vi "Accel calib routine.vi"(6 "Connection Status":T1={"MAC Address"="", "cnx handle"=0, "cnx flags"=0, "Address Type"=125, "Connection Interval (ms)"=125, "Timeout(ms)"=125, "Latency"=0, "bonding handle"=0} {"Address Type" items=["Public", "Random"]}, 8 "Error In":errorcluster, 11 "VISA resource in":refnum<visa-resource-name>) -> ()   [LabVIEW 2016]
uses:
  <vilib>/BLE/type_def/connection_status_bundle.ctl
  <vilib>/BLE/type_def/address_type.ctl
  Typedef/Accel calib - States.ctl
  Typedef/BLE char handle.ctl
  Typedef/Accel FSR.ctl
  <vilib>/Analysis/baseanly.llb/Mean (DBL).vi
  <vilib>/BLE/ble_functions/ble_write_by_handle_uint8array.vi
  <vilib>/Analysis/NI_AALBase.lvlib
panel:
  in  "Set & Save":bool
  in  "Exit":bool
  in  "Next":bool
  out "Calibration results":i32(listbox)
  out "Instructions":string="Press START CALIBRATION to calibrate the accelerometer"
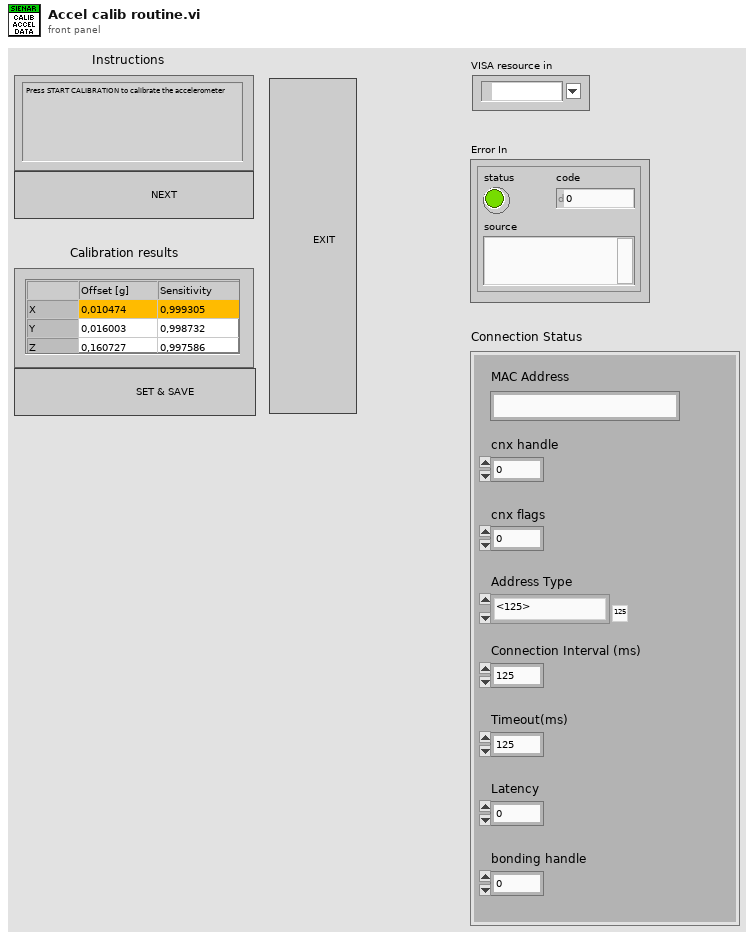
[diagram p1: front panel]
types:
  T1 = typedef "connection_status_bundle.ctl" = cluster{"MAC Address":string, "cnx handle":u8, "cnx flags":u8, "Address Type":T2, "Connection Interval (ms)":u16, "Timeout(ms)":u16, "Latency":u16, "bonding handle":u8}
  T2 = typedef "address_type.ctl" = u8
  T3 = typedef "Accel calib - States.ctl" = enum16{"Start calibration", "Acquire X+", "Acquire X-", "Acquire Y+", "Acquire Y-", "Acquire Z+", "Acquire Z-", "Display results", "Set & Save", "Exit"}
  T4 = typedef "Accel FSR.ctl" = enum16{"±2g", "±4g", "±8g", "±16g"}
  T5 = enum16{"Accelerometer", "Gyroscope", "Magnetometer"}
  T6 = typedef "BLE char handle.ctl" = u16
  T7 = cluster{"AccelData":cluster{"AccelX":i16, "AccelY":i16, "AccelZ":i16}, "GyroData":cluster{"GyroX":i16, "GyroY":i16, "GyroZ":i16}, "MagData":cluster{"MagX":i16, "MagY":i16, "MagZ":i16}}
  T8 = cluster{"AccelData":cluster{"AccelX":dbl, "AccelY":dbl, "AccelZ":dbl}, "GyroData":cluster{"GyroX":dbl, "GyroY":dbl, "GyroZ":dbl}, "MagData":cluster{"MagX":dbl, "MagY":dbl, "MagZ":dbl}}
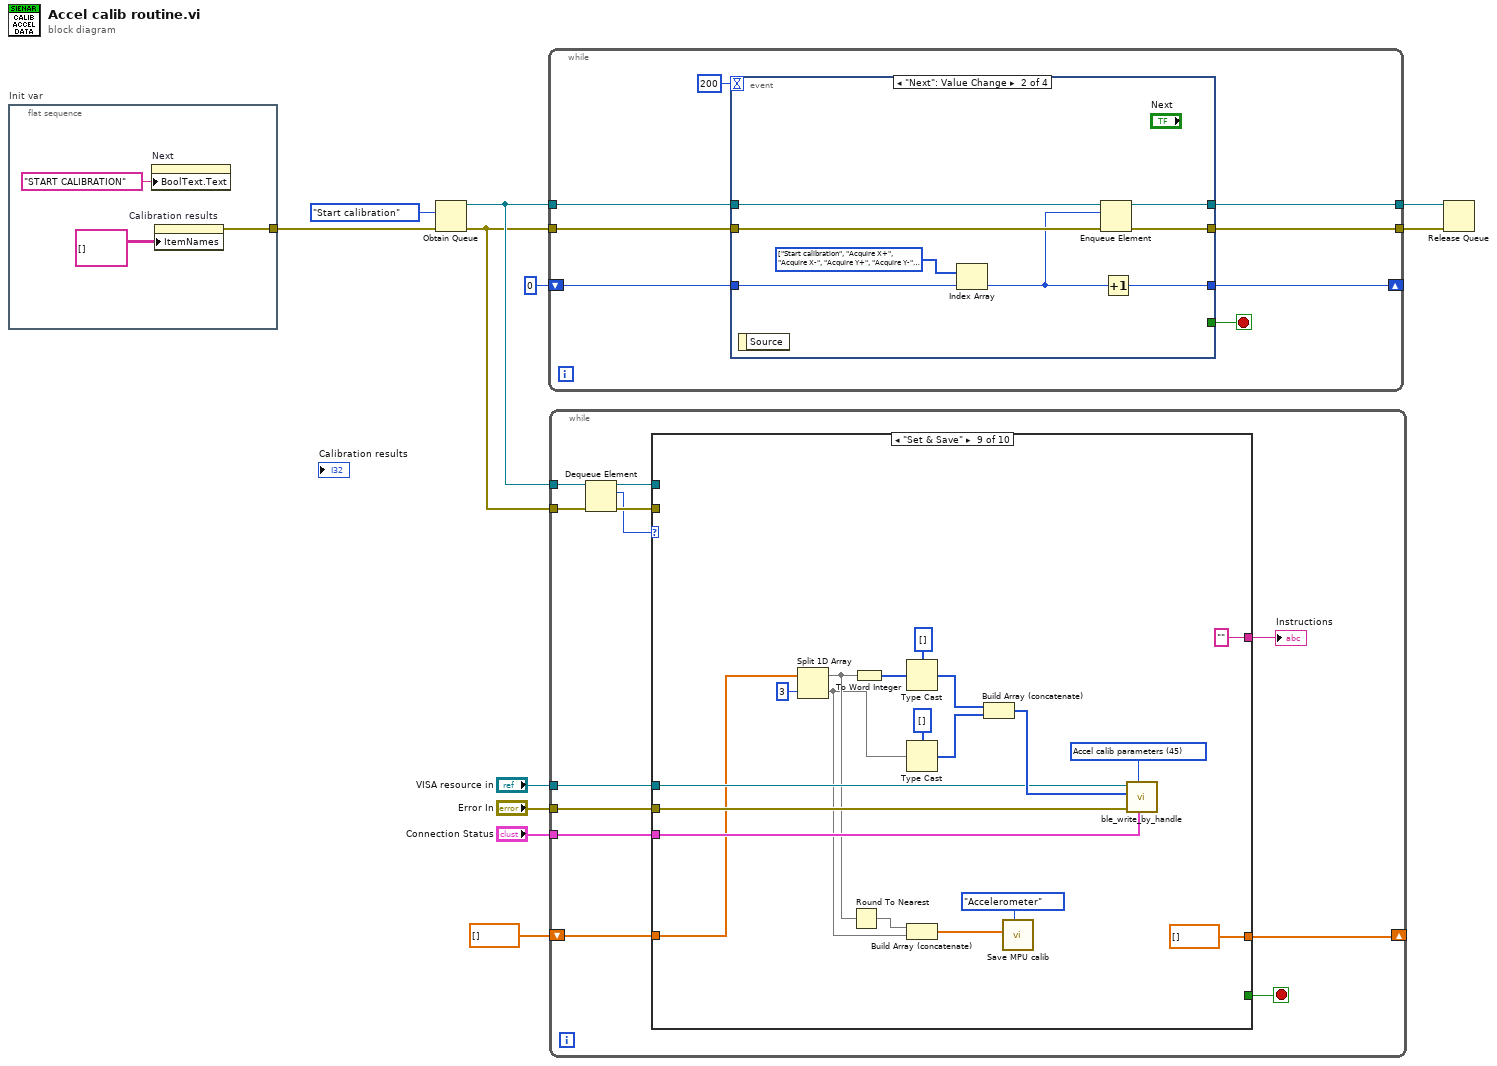
[diagram p0: block diagram]
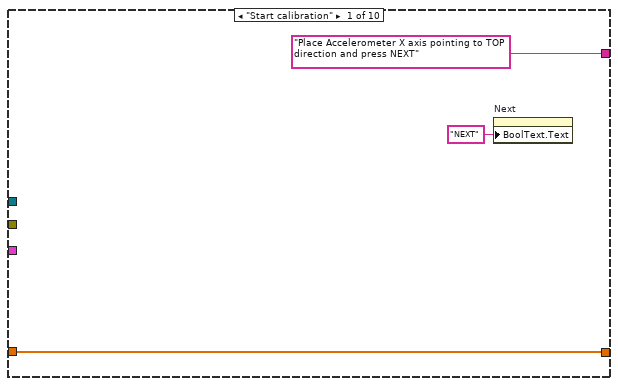
[diagram p2: hidden frame]
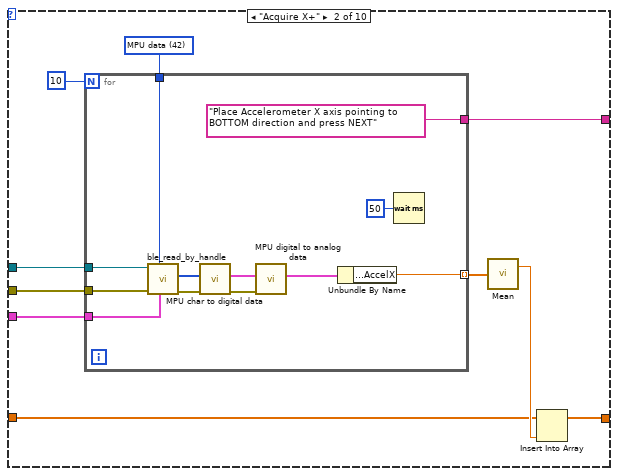
[diagram p3: hidden frame]
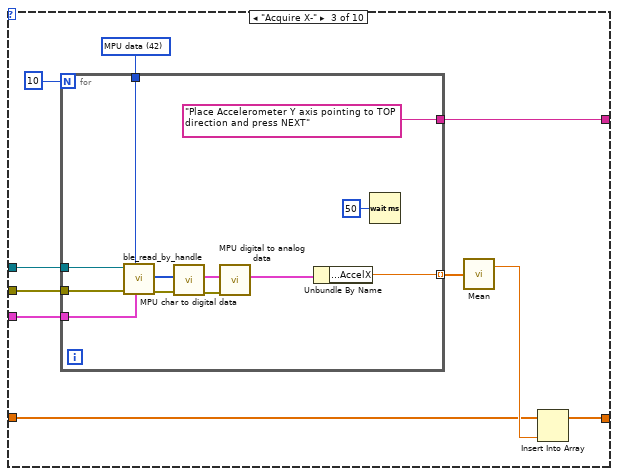
[diagram p4: hidden frame]
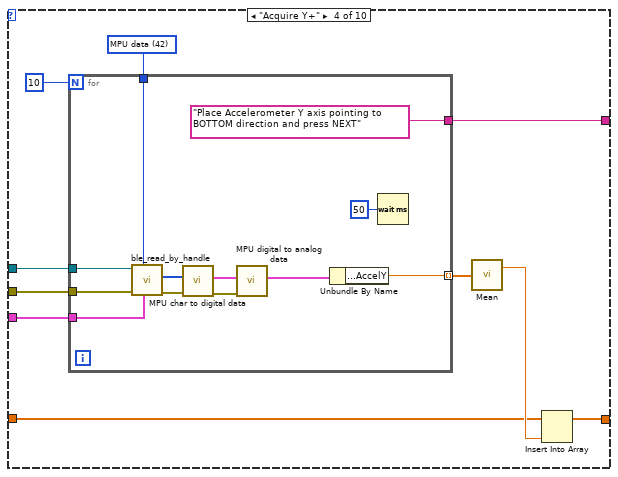
[diagram p5: hidden frame]
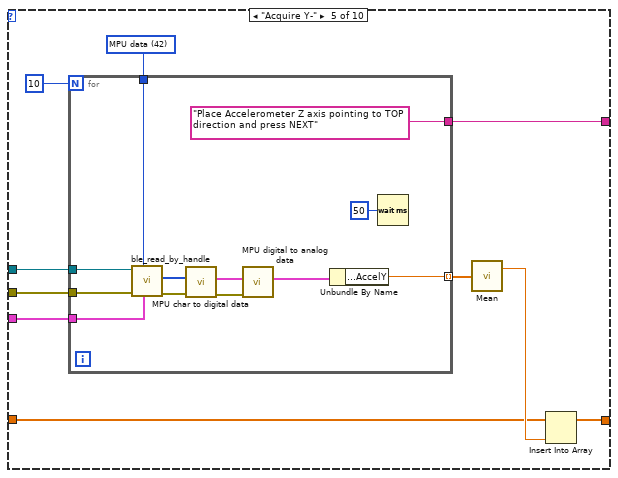
[diagram p6: hidden frame]
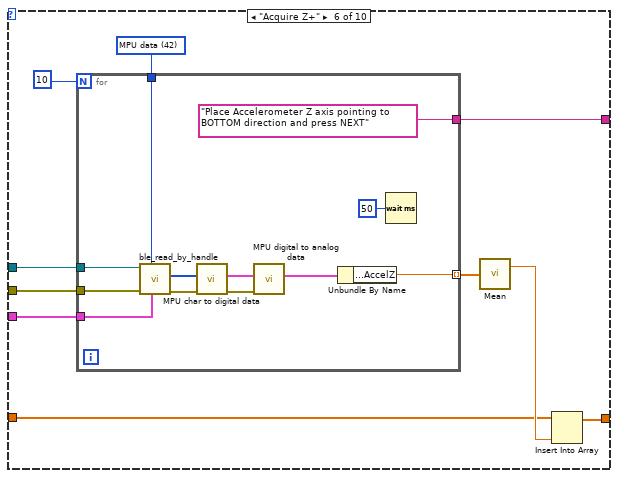
[diagram p7: hidden frame]
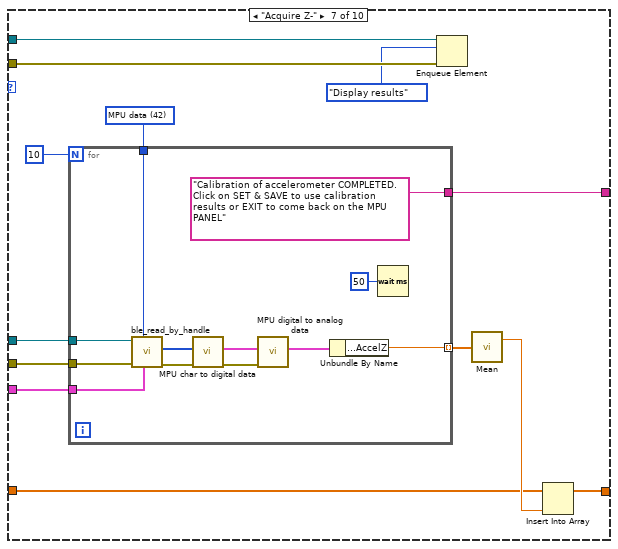
[diagram p8: hidden frame]
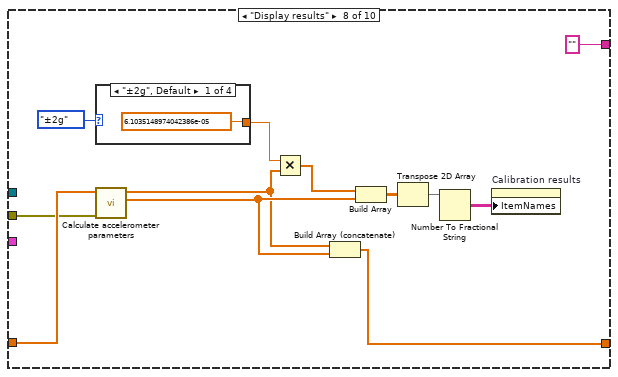
[diagram p9: hidden frame]
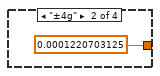
[diagram p10: hidden frame]
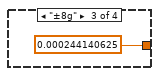
[diagram p11: hidden frame]
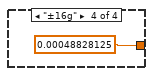
[diagram p12: hidden frame]
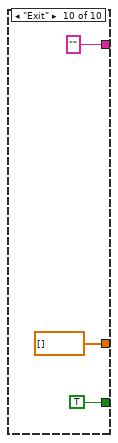
[diagram p13: hidden frame]
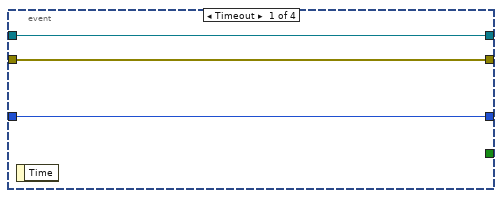
[diagram p14: hidden frame]
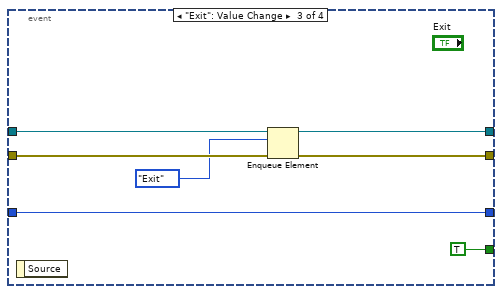
[diagram p15: hidden frame]
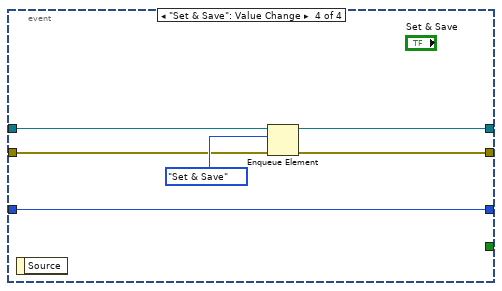
[diagram p16: hidden frame]
diagram:
  n1 = flat-sequence "Init var" {
    tunnel: [w13] -> w2
    frame #0 {
      n2 = property on="Next" class="Bool"("BoolText.Text"="START CALIBRATION" ("Boolean Text.Text")) -> ()  [unwired: 2 in, 2 out]
      n3 = property on="Calibration results" class="MCListbox (strict)"("ItemNames"=string[][] [] ("Item Names")) -> (error out=w13:errorcluster)  [unwired: 2 in, 1 out]
    }
  }
  n4 = Obtain Queue(element data type=Accel_calib_-_States."Start calibration", error in (no error)=w2) -> (queue out=w7:refnum<queue>, error out=w6:errorcluster)  [unwired: 3 in, 1 out]
  n5 = while {
    tunnel: w7 -> [w21]
    tunnel: w6 -> [w20]
    tunnel: [w19] -> w11
    tunnel: [w18] -> w10
    shift-right: [w16] -> _
    shift-left: 0 -> [w17]
    stop <- w15 stop-if-true
    n6 = event shown="[1] \"Next\": Value Change" {
      selector: _ -> [_ _ _ _]
      dyn-events: _ -> [_ _ _ _]
      timeout: 200 -> [_ _ _ _]
      tunnel: w21 -> [w25 w33 w40 w45]
      tunnel: w20 -> [w24 w32 w39 w44]
      tunnel: [w25 w31 w37 w41] -> w19
      tunnel: [w24 w30 w38 w42] -> w18
      tunnel: w17 -> [w23 w29 w35 w43]
      tunnel: [w23 w27 w35 w43] -> w16
      tunnel: [_ _ TRUE _] -> w15
      event Timeout {
        n7 = event-data() -> ()  [unwired: 1 in, 1 out]
      }
      event "Next": Value Change {
        w26 = T3[] [enum."Start calibration", enum."Acquire X+", enum."Acquire X-", enum."Acquire Y+", enum."Acquire Y-", enum."Acquire Z+", enum."Acquire Z-"] items=["Start calibration", "Acquire X+", "Acquire X-", "Acquire Y+", "Acquire Y-", "Acquire Z+", "Acquire Z-", "Display results", "Set & Save", "Exit"]
        n8 = event-data() -> ()  [unwired: 1 in, 1 out]
        n9 = Index Array(array=w26, index=w29) -> (element=w28:T3)
        n10 = Enqueue Element(queue=w33, element=w28, error in (no error)=w32) -> (queue out=w31:refnum<queue>, error out=w30:errorcluster)  [unwired: 1 in, 1 out]
        n11 = Increment(x=w28) -> (x+1=w27:T3)
      }
      event "Exit": Value Change {
        n12 = event-data() -> ()  [unwired: 1 in, 1 out]
        n13 = Enqueue Element(queue=w40, element=Accel_calib_-_States."Exit", error in (no error)=w39) -> (queue out=w37:refnum<queue>, error out=w38:errorcluster)  [unwired: 1 in, 1 out]
      }
      event "Set & Save": Value Change {
        n14 = event-data() -> ()  [unwired: 1 in, 1 out]
        n15 = Enqueue Element(queue=w45, element=Accel_calib_-_States."Set & Save", error in (no error)=w44) -> (queue out=w41:refnum<queue>, error out=w42:errorcluster)  [unwired: 1 in, 1 out]
      }
    }
  }
  n16 = while {
    tunnel: w7 -> [w58]
    tunnel: w6 -> [w57]
    tunnel: "VISA resource in" -> [w52]
    tunnel: "Error In" -> [w51]
    tunnel: "Connection Status" -> [w50]
    shift-right: [w47] -> _
    shift-left: sgl[] [] -> [w48]
    stop <- w49 stop-if-true
    n17 = Dequeue Element(queue=w58, error in (no error)=w57) -> (queue out=w56:refnum<queue>, element=w54:T3, error out=w55:errorcluster)  [unwired: 1 in, 1 out]
    n18 = case shown="\"Set & Save\"" w54 {
      tunnel: w56 -> [_ _ _ _ _ _ w179 _ _ _]
      tunnel: w55 -> [_ _ _ _ _ _ w178 _ _ _]
      tunnel: ["Place Accelerometer X axis pointing to TOP direction and press NEXT" ("message") w67 w89 w111 w133 w155 w180 "" ("message") "" ("message") "" ("message")] -> w53
      tunnel: w52 -> [_ w70 w92 w114 w136 w158 w183 _ w222 _]
      tunnel: w51 -> [_ w69 w91 w113 w135 w157 w182 w201 w221 _]
      tunnel: w50 -> [_ w68 w90 w112 w134 w156 w181 _ w220 _]
      tunnel: [_ _ _ _ _ _ _ _ _ TRUE] -> w49
      tunnel: w48 -> [w59 w64 w86 w108 w130 w152 w174 w203 w219 _]
      tunnel: [w59 w63 w85 w107 w129 w151 w173 w202 sgl[] [] sgl[] []] -> w47
      frame "Start calibration" {
        n19 = property on="Next" class="Bool"("BoolText.Text"="NEXT" ("Boolean Text.Text")) -> ()  [unwired: 2 in, 2 out]
      }
      frame "Acquire X+" {
        w62 = T6 42 items=["MPU data"=42, "MPU data - DESCR"=43, "Accel calib parameters"=45, "Gyro calib parameters"=47, "Mag calib parameters - 1"=49, "Mag calib parameters - 2"=51, "YPR"=53, "YPR - DESCR"=54, "Strain sensors"=56, "Strain sensors - DESCR"=57, "Wristband"=59, "Wristband - DESCR"=60] ("BLE char handle")
        n20 = for {
          N: 10 -> [_]
          tunnel: [w82] -> w65 mode=indexing
          tunnel: w62 -> [w81]
          tunnel: w70 -> [w80]
          tunnel: w69 -> [w79]
          tunnel: w68 -> [w78]
          tunnel: ["Place Accelerometer X axis pointing to BOTTOM direction and press NEXT" ("message")] -> w67
          n21 = call <vilib>:"ble_read_by_handle.vi"("Connection Status"=w78, "Handle"=w81, "error in (no error)"=w79, "COM Bluegiga in"=w80) -> ("error out"=w72:errorcluster, "characteristic value"=w73:u8[])  [unwired: 5 in, 1 out]
          n22 = call "MPU char to digital data.vi"("Error In"=w72, "MPU characteristic data"=w73) -> ("Error Out"=w76:errorcluster, "Digital MPU data"=w75:T7)  [unwired: 8 in]
          n23 = call "MPU digital to analog data.vi"("Error In"=w76, "Digital MPU data"=w75) -> ("Analog MPU data"=w74:T8)  [unwired: 8 in, 1 out]
          n24 = Unbundle By Name(w74) -> ("AccelData.AccelX"=w82:dbl)
          n25 = Wait (ms)(milliseconds to wait=u32 50) -> ()  [unwired: 1 out]
        }
        n26 = call-poly <vilib>:"Mean.vi"("X"=w65) -> ("mean"=w66:dbl)  [unwired: 1 out]
        n27 = Insert Into Array(array=w64, new element=w66) -> (w63:sgl[])  [unwired: 1 in]
      }
      frame "Acquire X-" {
        w84 = T6 42 items=["MPU data"=42, "MPU data - DESCR"=43, "Accel calib parameters"=45, "Gyro calib parameters"=47, "Mag calib parameters - 1"=49, "Mag calib parameters - 2"=51, "YPR"=53, "YPR - DESCR"=54, "Strain sensors"=56, "Strain sensors - DESCR"=57, "Wristband"=59, "Wristband - DESCR"=60] ("BLE char handle")
        n28 = for {
          N: 10 -> [_]
          tunnel: [w104] -> w87 mode=indexing
          tunnel: w84 -> [w103]
          tunnel: w92 -> [w102]
          tunnel: w91 -> [w101]
          tunnel: w90 -> [w100]
          tunnel: ["Place Accelerometer Y axis pointing to TOP direction and press NEXT" ("message")] -> w89
          n29 = call <vilib>:"ble_read_by_handle.vi"("Connection Status"=w100, "Handle"=w103, "error in (no error)"=w101, "COM Bluegiga in"=w102) -> ("error out"=w97:errorcluster, "characteristic value"=w98:u8[])  [unwired: 5 in, 1 out]
          n30 = call "MPU char to digital data.vi"("Error In"=w97, "MPU characteristic data"=w98) -> ("Error Out"=w95:errorcluster, "Digital MPU data"=w96:T7)  [unwired: 8 in]
          n31 = call "MPU digital to analog data.vi"("Error In"=w95, "Digital MPU data"=w96) -> ("Analog MPU data"=w94:T8)  [unwired: 8 in, 1 out]
          n32 = Unbundle By Name(w94) -> ("AccelData.AccelX"=w104:dbl)
          n33 = Wait (ms)(milliseconds to wait=u32 50) -> ()  [unwired: 1 out]
        }
        n34 = call-poly <vilib>:"Mean.vi"("X"=w87) -> ("mean"=w88:dbl)  [unwired: 1 out]
        n35 = Insert Into Array(array=w86, new element=w88) -> (w85:sgl[])  [unwired: 1 in]
      }
      frame "Acquire Y+" {
        w106 = T6 42 items=["MPU data"=42, "MPU data - DESCR"=43, "Accel calib parameters"=45, "Gyro calib parameters"=47, "Mag calib parameters - 1"=49, "Mag calib parameters - 2"=51, "YPR"=53, "YPR - DESCR"=54, "Strain sensors"=56, "Strain sensors - DESCR"=57, "Wristband"=59, "Wristband - DESCR"=60] ("BLE char handle")
        n36 = for {
          N: 10 -> [_]
          tunnel: [w126] -> w109 mode=indexing
          tunnel: w106 -> [w125]
          tunnel: w114 -> [w124]
          tunnel: w113 -> [w123]
          tunnel: w112 -> [w122]
          tunnel: ["Place Accelerometer Y axis pointing to BOTTOM direction and press NEXT" ("message")] -> w111
          n37 = call <vilib>:"ble_read_by_handle.vi"("Connection Status"=w122, "Handle"=w125, "error in (no error)"=w123, "COM Bluegiga in"=w124) -> ("error out"=w119:errorcluster, "characteristic value"=w120:u8[])  [unwired: 5 in, 1 out]
          n38 = call "MPU char to digital data.vi"("Error In"=w119, "MPU characteristic data"=w120) -> ("Error Out"=w118:errorcluster, "Digital MPU data"=w117:T7)  [unwired: 8 in]
          n39 = call "MPU digital to analog data.vi"("Error In"=w118, "Digital MPU data"=w117) -> ("Analog MPU data"=w116:T8)  [unwired: 8 in, 1 out]
          n40 = Unbundle By Name(w116) -> ("AccelData.AccelY"=w126:dbl)
          n41 = Wait (ms)(milliseconds to wait=u32 50) -> ()  [unwired: 1 out]
        }
        n42 = call-poly <vilib>:"Mean.vi"("X"=w109) -> ("mean"=w110:dbl)  [unwired: 1 out]
        n43 = Insert Into Array(array=w108, new element=w110) -> (w107:sgl[])  [unwired: 1 in]
      }
      frame "Acquire Y-" {
        w128 = T6 42 items=["MPU data"=42, "MPU data - DESCR"=43, "Accel calib parameters"=45, "Gyro calib parameters"=47, "Mag calib parameters - 1"=49, "Mag calib parameters - 2"=51, "YPR"=53, "YPR - DESCR"=54, "Strain sensors"=56, "Strain sensors - DESCR"=57, "Wristband"=59, "Wristband - DESCR"=60] ("BLE char handle")
        n44 = for {
          N: 10 -> [_]
          tunnel: [w148] -> w131 mode=indexing
          tunnel: w128 -> [w147]
          tunnel: w136 -> [w146]
          tunnel: w135 -> [w145]
          tunnel: w134 -> [w144]
          tunnel: ["Place Accelerometer Z axis pointing to TOP direction and press NEXT" ("message")] -> w133
          n45 = call <vilib>:"ble_read_by_handle.vi"("Connection Status"=w144, "Handle"=w147, "error in (no error)"=w145, "COM Bluegiga in"=w146) -> ("error out"=w141:errorcluster, "characteristic value"=w142:u8[])  [unwired: 5 in, 1 out]
          n46 = call "MPU char to digital data.vi"("Error In"=w141, "MPU characteristic data"=w142) -> ("Error Out"=w139:errorcluster, "Digital MPU data"=w140:T7)  [unwired: 8 in]
          n47 = call "MPU digital to analog data.vi"("Error In"=w139, "Digital MPU data"=w140) -> ("Analog MPU data"=w138:T8)  [unwired: 8 in, 1 out]
          n48 = Unbundle By Name(w138) -> ("AccelData.AccelY"=w148:dbl)
          n49 = Wait (ms)(milliseconds to wait=u32 50) -> ()  [unwired: 1 out]
        }
        n50 = call-poly <vilib>:"Mean.vi"("X"=w131) -> ("mean"=w132:dbl)  [unwired: 1 out]
        n51 = Insert Into Array(array=w130, new element=w132) -> (w129:sgl[])  [unwired: 1 in]
      }
      frame "Acquire Z+" {
        w150 = T6 42 items=["MPU data"=42, "MPU data - DESCR"=43, "Accel calib parameters"=45, "Gyro calib parameters"=47, "Mag calib parameters - 1"=49, "Mag calib parameters - 2"=51, "YPR"=53, "YPR - DESCR"=54, "Strain sensors"=56, "Strain sensors - DESCR"=57, "Wristband"=59, "Wristband - DESCR"=60] ("BLE char handle")
        n52 = for {
          N: 10 -> [_]
          tunnel: [w170] -> w153 mode=indexing
          tunnel: w150 -> [w169]
          tunnel: w158 -> [w168]
          tunnel: w157 -> [w167]
          tunnel: w156 -> [w166]
          tunnel: ["Place Accelerometer Z axis pointing to BOTTOM direction and press NEXT" ("message")] -> w155
          n53 = call <vilib>:"ble_read_by_handle.vi"("Connection Status"=w166, "Handle"=w169, "error in (no error)"=w167, "COM Bluegiga in"=w168) -> ("error out"=w164:errorcluster, "characteristic value"=w163:u8[])  [unwired: 5 in, 1 out]
          n54 = call "MPU char to digital data.vi"("Error In"=w164, "MPU characteristic data"=w163) -> ("Error Out"=w161:errorcluster, "Digital MPU data"=w162:T7)  [unwired: 8 in]
          n55 = call "MPU digital to analog data.vi"("Error In"=w161, "Digital MPU data"=w162) -> ("Analog MPU data"=w160:T8)  [unwired: 8 in, 1 out]
          n56 = Unbundle By Name(w160) -> ("AccelData.AccelZ"=w170:dbl)
          n57 = Wait (ms)(milliseconds to wait=u32 50) -> ()  [unwired: 1 out]
        }
        n58 = call-poly <vilib>:"Mean.vi"("X"=w153) -> ("mean"=w154:dbl)  [unwired: 1 out]
        n59 = Insert Into Array(array=w152, new element=w154) -> (w151:sgl[])  [unwired: 1 in]
      }
      frame "Acquire Z-" {
        w172 = T6 42 items=["MPU data"=42, "MPU data - DESCR"=43, "Accel calib parameters"=45, "Gyro calib parameters"=47, "Mag calib parameters - 1"=49, "Mag calib parameters - 2"=51, "YPR"=53, "YPR - DESCR"=54, "Strain sensors"=56, "Strain sensors - DESCR"=57, "Wristband"=59, "Wristband - DESCR"=60] ("BLE char handle")
        n60 = for {
          N: 10 -> [_]
          tunnel: [w195] -> w175 mode=indexing
          tunnel: w172 -> [w194]
          tunnel: w183 -> [w193]
          tunnel: w182 -> [w192]
          tunnel: w181 -> [w191]
          tunnel: ["Calibration of accelerometer COMPLETED. Click on SET & SAVE to use calibration results or EXIT to come back on the MPU PANEL" ("message")] -> w180
          n61 = call <vilib>:"ble_read_by_handle.vi"("Connection Status"=w191, "Handle"=w194, "error in (no error)"=w192, "COM Bluegiga in"=w193) -> ("error out"=w188:errorcluster, "characteristic value"=w189:u8[])  [unwired: 5 in, 1 out]
          n62 = call "MPU char to digital data.vi"("Error In"=w188, "MPU characteristic data"=w189) -> ("Error Out"=w187:errorcluster, "Digital MPU data"=w186:T7)  [unwired: 8 in]
          n63 = call "MPU digital to analog data.vi"("Error In"=w187, "Digital MPU data"=w186) -> ("Analog MPU data"=w185:T8)  [unwired: 8 in, 1 out]
          n64 = Unbundle By Name(w185) -> ("AccelData.AccelZ"=w195:dbl)
          n65 = Wait (ms)(milliseconds to wait=u32 50) -> ()  [unwired: 1 out]
        }
        n66 = Enqueue Element(queue=w179, element=Accel_calib_-_States."Display results", error in (no error)=w178) -> ()  [unwired: 1 in, 3 out]
        n67 = call-poly <vilib>:"Mean.vi"("X"=w175) -> ("mean"=w176:dbl)  [unwired: 1 out]
        n68 = Insert Into Array(array=w174, new element=w176) -> (w173:sgl[])  [unwired: 1 in]
      }
      frame "Display results" {
        n69 = case shown="\"±2g\", Default" Accel_FSR."±2g" ("Accel FSR") {
          tunnel: [sgl 6.103515e-05 sgl 0.00012207031 sgl 0.00024414062 sgl 0.00048828125] -> w198
          frame "±2g", Default {
          }
          frame "±4g" {
          }
          frame "±8g" {
          }
          frame "±16g" {
          }
        }
        n70 = call "Calculate accelerometer parameters.vi"("Error In"=w201, "Data in"=w203) -> ("Accel Sensitivities"=w206:sgl[], "Accel Offset"=w199:sgl[])  [unwired: 7 in, 1 out]
        n71 = Multiply(x=w198, y=w199) -> (x*y=w197:sgl[])
        n72 = Build Array (concatenate)(w199, w206) -> (w202:sgl[])
        n73 = Build Array(w197, w206) -> (w205:sgl[][])
        n74 = Transpose 2D Array(2D array=w205) -> (transposed array=w204:sgl[][])
        n75 = Number To Fractional String(number=w204) -> (F-format string=w207:string[][])  [unwired: 3 in]
        n76 = property on="Calibration results" class="MCListbox (strict)"("ItemNames"=w207) -> ()  [unwired: 2 in, 2 out]
      }
      frame "Set & Save" {
        w213 = T6 45 items=["MPU data"=42, "MPU data - DESCR"=43, "Accel calib parameters"=45, "Gyro calib parameters"=47, "Mag calib parameters - 1"=49, "Mag calib parameters - 2"=51, "YPR"=53, "YPR - DESCR"=54, "Strain sensors"=56, "Strain sensors - DESCR"=57, "Wristband"=59, "Wristband - DESCR"=60] ("BLE char handle")
        n77 = Split 1D Array(array=w219, index=3) -> (first subarray=w216:sgl[], second subarray=w215:sgl[])
        n78 = Round To Nearest(number=w216) -> (nearest integer value=w217:sgl[])
        n79 = To Word Integer(number=w216) -> (16bit integer=w228:i16[])
        n80 = Type Cast(type=u8[] [], x=w228) -> (*(type *) &x=w225:u8[])
        n81 = Type Cast(type=u8[] [], x=w215) -> (*(type *) &x=w224:u8[])
        n82 = Build Array (concatenate)(w217, w215) -> (w214:sgl[])
        n83 = Build Array (concatenate)(w225, w224) -> (w223:u8[])
        n84 = call "Save MPU calib.vi"("Calib data type"=T5."Accelerometer", "Calib data"=w214) -> ()  [unwired: 9 in, 1 out]
        n85 = call-poly <vilib>:"ble_write_by_handle.vi"("Connection Status"=w220, "Handle"=w213, "error in (no error)"=w221, "data (uint8array)"=w223, "COM Bluegiga in"=w222) -> ()  [unwired: 5 in, 2 out]
      }
      frame "Exit" {
      }
    }
    "Instructions" <- w53
  }
  n86 = Release Queue(queue=w11, error in (no error)=w10) -> ()  [unwired: 1 in, 3 out]
